vi "Default Serial Port Configuration--constant.vi"(11 "Port":string) -> (3 "Serial Port Config":T1 {"Bits per second (baud rate)" items=["4800"=4800, "9600"=9600, "14400"=14400, "19200"=19200, "38400"=38400, "57600"=57600, "115200"=115200, "128000"=128000, "230400"=230400]; "Stop bits" items=["1.0"=10, "1.5"=15, "2.0"=20]; "Flow control" items=["None", "XON/XOFF", "RTS/CTS", "XON/XOFF & RTS/CTS", "DTR/DSR", "XON/XOFF & DTR/DSR"]})   [LabVIEW 2017, in "Serial Device.lvclass"]
doc: "This VI holds the default configuration constants.\nThe Timeout is calculated to be a second less than the module's timeout, so the serial error time out is received before a Request and Wait for Reply DQMH event time out."
uses:
  Serial Device.lvclass
  Serial Port configuration--cluster.ctl
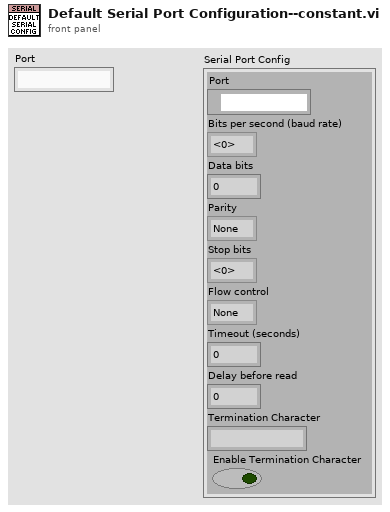
[diagram p1: front panel]
types:
  T1 = typedef "Serial Device.lvclass/Serial Port configuration--cluster.ctl" = cluster{"Port":refnum<visa-resource-name>, "Bits per second (baud rate)":u32, "Data bits":u16, "Parity":enum16{"None", "Odd", "Even", "Mark", "Space"}, "Stop bits":u16, "Flow control":u16, "Timeout (seconds)":u32, "Delay before read":dbl, "Termination Character":string, "Enable Termination Character":bool}
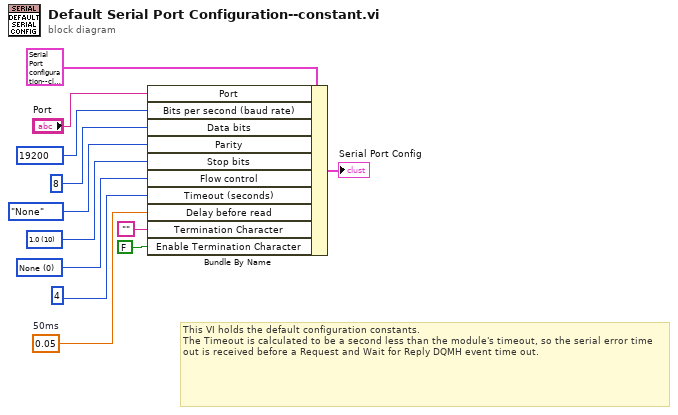
[diagram p0: block diagram]
diagram:
  w12 = u16 10 items=["1.0"=10, "1.5"=15, "2.0"=20] ("Stop bits")
  w9 = u16 0 items=["None", "XON/XOFF", "RTS/CTS", "XON/XOFF & RTS/CTS", "DTR/DSR", "XON/XOFF & DTR/DSR"] ("Flow control")
  w4 = 0.05  # 50ms
  w6 = u32 19200 items=["4800"=4800, "9600"=9600, "14400"=14400, "19200"=19200, "38400"=38400, "57600"=57600, "115200"=115200, "128000"=128000, "230400"=230400] ("Bits per second (baud rate)")
  # "This VI holds the default configuration constants.\nThe Timeout is calculated to be a second less than the module's timeout, so the serial error time out is received before a Request and Wait for Reply DQMH event time out."
  n1 = Bundle By Name(cluster=T1 {"Port"="", "Bits per second (baud rate)"=115200, "Data bits"=8, "Parity"=enum."None", "Stop bits"=10, "Flow control"=0, "Timeout (seconds)"=10, "Delay before read"=0.5, "Termination Character"="\\r\\n", "Enable Termination Character"=TRUE} ("Serial Port Config"), "Port"="Port", "Bits per second (baud rate)"=w6, "Data bits"=u16 8, "Parity"=enum16{"None", "Odd", "Even", "Mark", "Space"}."None", "Stop bits"=w12, "Flow control"=w9, "Timeout (seconds)"=4 ("y"), "Delay before read"=w4, "Termination Character"="", "Enable Termination Character"=FALSE) -> (→"Serial Port Config":T1)
